vi "Set Channel Count.vi"(10 "channel count":u64, 11 "DBL Buffer in":refnum<class "Double Pointer.lvclass">) -> (3 "DBL Buffer out":refnum<class "Double Pointer.lvclass">)   [LabVIEW 2017, in "Data Sharing Framework Engine.lvlib" / "Double Pointer.lvclass"]
uses:
  Double Pointer.lvclass
  Double Pointer.lvclass/Double Pointer.ctl
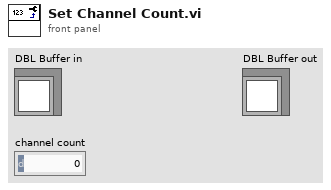
[diagram p1: front panel]
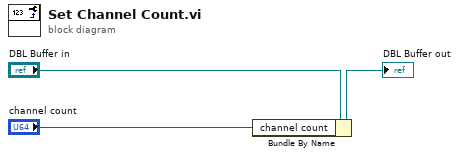
[diagram p0: block diagram]
diagram:
  n1 = Bundle By Name(cluster="DBL Buffer in", "channel count"="channel count") -> (→"DBL Buffer out":refnum<class "Double Pointer.lvclass">)
